vi "ScopeGUI.vi"() -> ()   [LabVIEW 2019]
uses:
  Scope Driver/Typedef/TimeSetting.ctl
  Scope Driver/Typedef/RangeSetting.ctl
  Typedef/Message Format.ctl
  Typedef/Scope Action.ctl
  Typedef/Consumer Loop Data.ctl
  Scope Driver/Typedef/Vertical Settings.ctl
  Scope Driver/Typedef/Channel Selection.ctl
  Scope Driver/Typedef/Coupling.ctl
  Scope Driver/Typedef/TriggerData.ctl
  Scope Driver/Typedef/Edge.ctl
  Scope Driver/Typedef/Horizontal Settings.ctl
  Scope Driver/Typedef/Metadata/[Meta]SetupInfoH.ctl
  Scope Driver/Typedef/Metadata/[Meta]SetupInfoV.ctl
  Scope Driver/Typedef/Metadata/[Meta]SetupInfoTrigger.ctl
  C:/Program Files (x86)/LabNation/SmartScope/DeviceInterface.dll
  Program Files (x86)/LabNation/SmartScope/DeviceInterface.dll
  Scope Driver/LabNation Scope Driver.lvlib
panel:
  in  "Connect":bool
  in  "Tab Control":enum32{"Waveform", "XY"}(tab)
  out "Scope Display":dbl[][](graph)
  in  "Trigger Level":dbl(slide) scale=-4.0..4.0
  in  "Trigger Hold Off":dbl(slide) scale=-2.5e-05..2.5e-05
  out "XY Graph":T1(graph)
  in  "Stop":bool
  in  "ChB Offset":dbl(slide) scale=-4.0..4.0
  in  "ChB V/div":T2=1.0 caption="Knob" scale=0.02..5.0
  in  "ChA Offset":dbl(slide) scale=-4.0..4.0
  in  "ChA V/div":T2=1.0 caption="Knob" scale=0.02..5.0
  out "Connected":bool
  in  "Time/div":T3=0.01 scale=0.0001..1.0 scale format="%#_8g"
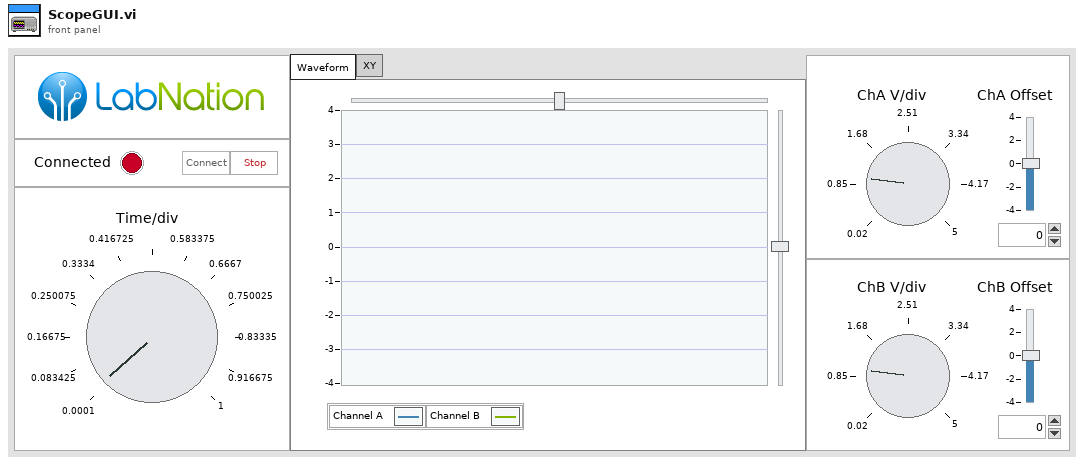
[diagram p1: front panel]
types:
  T1 = cluster{"Waveform Graph":dbl[], "Waveform Graph":dbl[]}
  T2 = typedef "LabNation Scope Driver.lvlib/RangeSetting.ctl" = dbl
  T3 = typedef "LabNation Scope Driver.lvlib/TimeSetting.ctl" = dbl
  T4 = typedef "Message Format.ctl" = cluster{"Action":T5, "Data":variant}
  T5 = typedef "Scope Action.ctl" = enum16{"--- Driver Functions ---", "Init", "SetupV", "SetupTrigger", "SetupH", "AcquireData", "--- UI Setup ---", "UIGraphH", "UIGraphV", "UITrigger", "--- Program Flow ---", "Error Handling", "Stop"}
  T6 = typedef "Consumer Loop Data.ctl" = cluster{"reference":refnum<k24>, "user event out":refnum<user-event>, "Connected?":bool}
  T7 = enum8{"Enabled", "Disabled", "Disabled and Grayed Out"}
  T8 = typedef "LabNation Scope Driver.lvlib/Vertical Settings.ctl" = cluster{"ChannelSelection":T9, "Coupling":T10, "Offset[V]":dbl, "V/div":T2}
  T9 = typedef "LabNation Scope Driver.lvlib/Channel Selection.ctl" = enum16{"chn A", "chn B"}
  T10 = typedef "LabNation Scope Driver.lvlib/Coupling.ctl" = i32
  T11 = typedef "LabNation Scope Driver.lvlib/TriggerData.ctl" = cluster{"Channel":T9, "Edge":T12, "Level[V]":sgl}
  T12 = typedef "LabNation Scope Driver.lvlib/Edge.ctl" = i32
  T13 = typedef "LabNation Scope Driver.lvlib/Horizontal Settings.ctl" = cluster{"Time/div":T3, "Trigger Holdoff":dbl}
  T14 = typedef "LabNation Scope Driver.lvlib/[Meta]SetupInfoH.ctl" = cluster{"xBegin":dbl, "xEnd":dbl}
  T15 = typedef "LabNation Scope Driver.lvlib/[Meta]SetupInfoV.ctl" = cluster{"ChannelSelection":T9, "GraphMin":dbl, "GraphMax":dbl, "OffsetMin":dbl, "OffsetMax":dbl}
  T16 = typedef "LabNation Scope Driver.lvlib/[Meta]SetupInfoTrigger.ctl" = cluster{"Trigger Maximum":dbl, "Trigger Minimum":dbl}
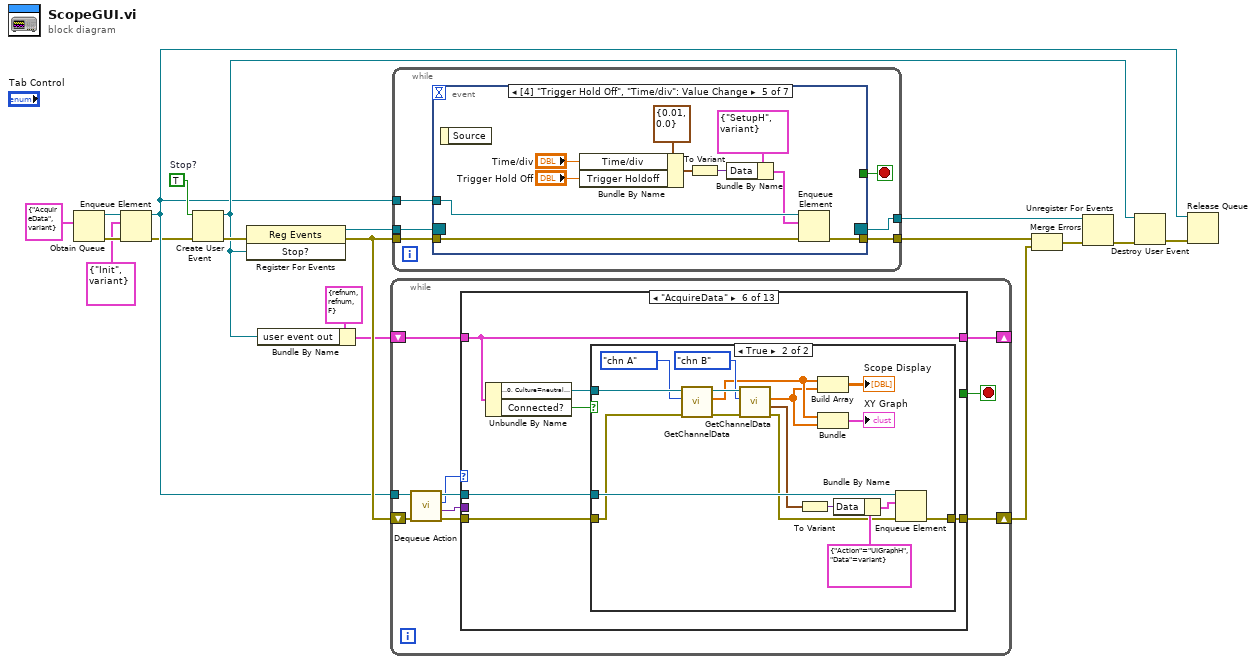
[diagram p0: block diagram]
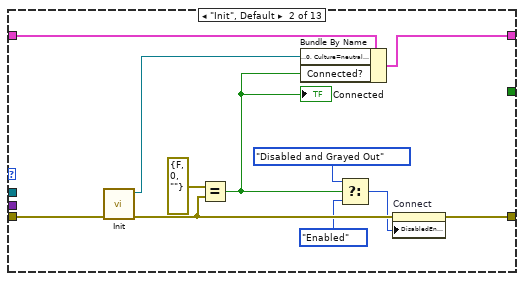
[diagram p3: hidden frame]
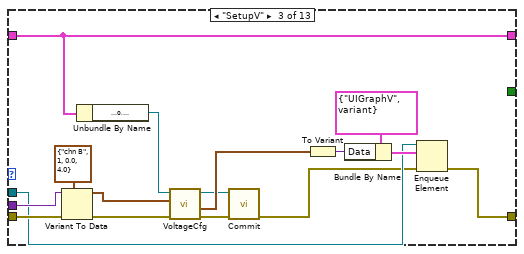
[diagram p4: hidden frame]
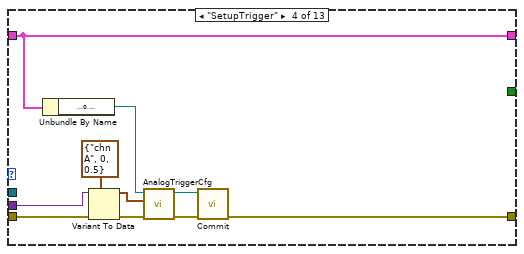
[diagram p5: hidden frame]
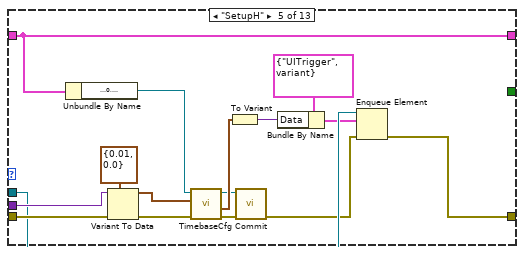
[diagram p6: hidden frame]
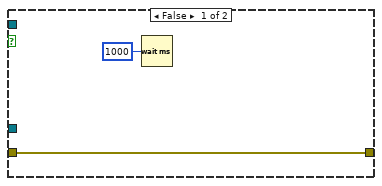
[diagram p7: hidden frame]
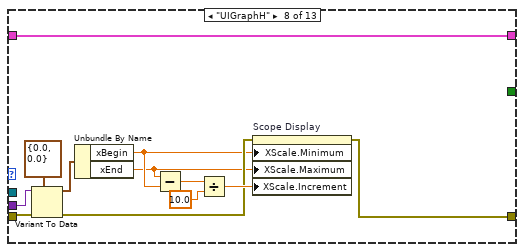
[diagram p9: hidden frame]
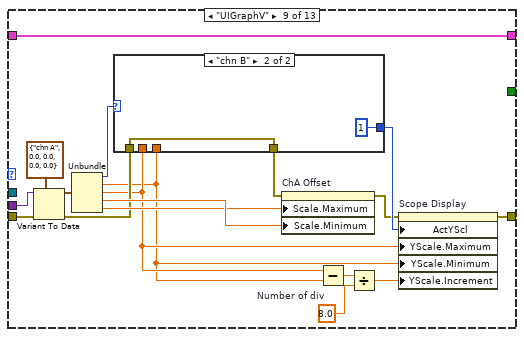
[diagram p10: hidden frame]
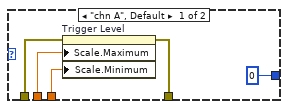
[diagram p11: hidden frame]
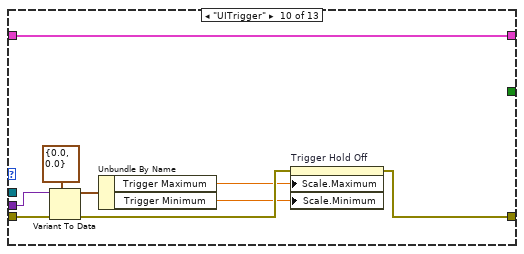
[diagram p12: hidden frame]
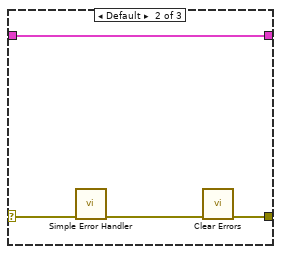
[diagram p15: hidden frame]
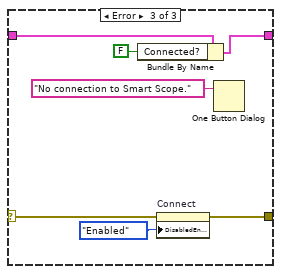
[diagram p16: hidden frame]
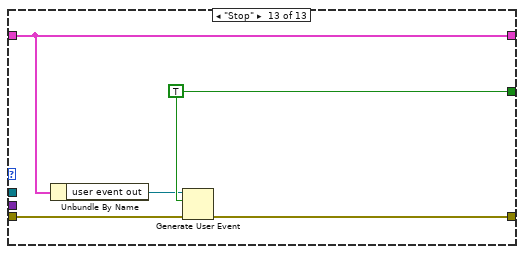
[diagram p17: hidden frame]
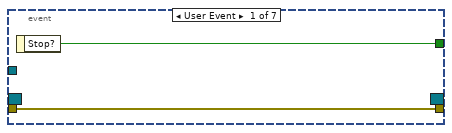
[diagram p18: hidden frame]
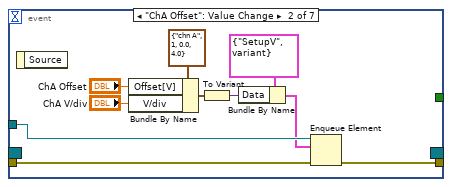
[diagram p19: hidden frame]
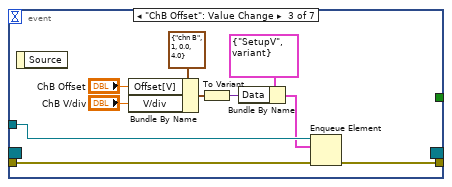
[diagram p20: hidden frame]
diagram:
  w18 = TRUE  # Stop?
  n1 = Obtain Queue(element data type=T4 {"Action"=enum."AcquireData", "Data"=variant}) -> (queue out=w5:refnum<queue>, error out=w2:errorcluster)  [unwired: 4 in, 1 out]
  n2 = Enqueue Element(queue=w5, element=T4 {"Action"=enum."Init", "Data"=variant}, error in (no error)=w2) -> (queue out=w4:refnum<queue>, error out=w3:errorcluster)  [unwired: 1 in, 1 out]
  n3 = Create User Event(user event datatype=w18, error in=w3) -> (user event=w7:refnum<user-event>, error out=w17:errorcluster)
  n4 = register-events(error in=w17, w7) -> (reference out=w19:refnum<event-registration>, error out=w10:errorcluster)  [unwired: 1 in]
  n5 = Bundle By Name(cluster=T6 {"reference"=refnum, "user event out"=refnum, "Connected?"=FALSE}, "user event out"=w7) -> (w6:T6)
  n6 = while {
    tunnel: w4 -> [w28]
    shift-right: [w24] -> w9
    shift-left: w10 -> [w29]
    shift-right: [w21] -> _
    shift-left: w6 -> [w22]
    stop <- w23 stop-if-true
    n7 = call "Dequeue Action.vi"("error in (no error)"=w29, "Queue in"=w28) -> ("error out"=w25:errorcluster, "Data"=w20:variant, "Action"=w26:T5, "Queue out"=w27:refnum<queue>)  [unwired: 6 in]
    n8 = case shown="\"AcquireData\"" w26 {
      tunnel: w27 -> [_ _ w45 _ w75 w86 _ _ _ _ _ _ _]
      tunnel: w20 -> [_ _ w53 w63 w80 _ _ w119 w139 w154 _ _ _]
      tunnel: w25 -> [w30 w42 w58 w68 w81 w90 w110 w121 w140 w157 w158 w162 w181]
      tunnel: w22 -> [w31 w41 w56 w65 w84 w88 w111 w112 w141 w149 w159 w160 w177]
      tunnel: [w30 w36 w46 w60 w74 w87 w110 w116 w132 w155 w158 w163 w180] -> w24
      tunnel: [_ _ _ _ _ _ _ _ _ _ _ _ w179] -> w23
      tunnel: [w31 w40 w56 w65 w84 w88 w111 w112 w141 w149 w159 w161 w177] -> w21
      frame "--- Driver Functions ---" {
      }
      frame "Init", Default {
        n9 = call "Init.vi"("error in (no error)"=w42) -> ("error out"=w37:errorcluster, "reference out"=w39:refnum<k24>)  [unwired: 9 in]
        n10 = Equal?(x=errorcluster {"status"=FALSE, "code"=0, "source"=""}, y=w37) -> (x = y?=w35:bool)
        "Connected" <- w35
        n11 = Bundle By Name(cluster=w41, "reference"=w39, "Connected?"=w35) -> (w40:T6)
        n12 = Select(t=T7."Disabled and Grayed Out" ("Disabled"), s=w35, f=T7."Enabled" ("Disabled")) -> (s? t:f=w32:T7)
        n13 = property on="Connect" class="Bool"(error in=w37, "DisabledEnum"=w32) -> (error out=w36:errorcluster)  [unwired: 1 in, 1 out]
      }
      frame "SetupV" {
        n14 = Variant To Data(error in=w58, type=T8 {"ChannelSelection"=enum."chn B", "Coupling"=1, "Offset[V]"=0.0, "V/div"=4.0} ("Vertical Settings"), Variant=w53) -> (data=w52:T8, error out=w55:errorcluster)
        n15 = Unbundle By Name(w56) -> ("reference"=w57:refnum<k24>)
        n16 = call "VoltageCfg.vi"("error in (no error)"=w55, "Vertical Settings"=w52, "reference in"=w57) -> ("error out"=w47:errorcluster, "Setup Info Vertical"=w48:T15, "reference out"=w43:refnum<k24>)  [unwired: 6 in]
        n17 = call "Commit.vi"("error in (no error)"=w47, "reference in"=w43) -> ("error out"=w44:errorcluster)  [unwired: 8 in, 1 out]
        n18 = To Variant(anything=w48) -> (Variant=w51:variant)
        n19 = Bundle By Name(cluster=T4 {"Action"=enum."UIGraphV", "Data"=variant} ("element"), "Data"=w51) -> (w50:T4)
        n20 = Enqueue Element(queue=w45, element=w50, error in (no error)=w44) -> (error out=w46:errorcluster)  [unwired: 1 in, 2 out]
      }
      frame "SetupTrigger" {
        n21 = Unbundle By Name(w65) -> ("reference"=w66:refnum<k24>)
        n22 = Variant To Data(error in=w68, type=T11 {"Channel"=enum."chn A", "Edge"=0, "Level[V]"=0.5} ("Trigger Config"), Variant=w63) -> (data=w61:T11, error out=w64:errorcluster)
        n23 = call "AnalogTriggerCfg.vi"("error in (no error)"=w64, "Trigger Config"=w61, "reference in"=w66) -> ("error out"=w67:errorcluster, "reference out"=w59:refnum<k24>)  [unwired: 7 in]
        n24 = call "Commit.vi"("error in (no error)"=w67, "reference in"=w59) -> ("error out"=w60:errorcluster)  [unwired: 8 in, 1 out]
      }
      frame "SetupH" {
        n25 = Unbundle By Name(w84) -> ("reference"=w83:refnum<k24>)
        n26 = Variant To Data(error in=w81, type=T13 {"Time/div"=0.01, "Trigger Holdoff"=0.0} ("Horizontal Settings"), Variant=w80) -> (data=w78:T13, error out=w82:errorcluster)
        n27 = call "TimebaseCfg.vi"("error in (no error)"=w82, "Horizontal Settings"=w78, "reference in"=w83) -> ("error out"=w76:errorcluster, "Setup Info Horizontal"=w77:T16, "reference out"=w69:refnum<k24>)  [unwired: 6 in]
        n28 = To Variant(anything=w77) -> (Variant=w71:variant)
        n29 = call "Commit.vi"("error in (no error)"=w76, "reference in"=w69) -> ("error out"=w70:errorcluster)  [unwired: 8 in, 1 out]
        n30 = Bundle By Name(cluster=T4 {"Action"=enum."UITrigger", "Data"=variant} ("element"), "Data"=w71) -> (w72:T4)
        n31 = Enqueue Element(queue=w75, element=w72, error in (no error)=w70) -> (error out=w74:errorcluster)  [unwired: 1 in, 2 out]
      }
      frame "AcquireData" {
        n32 = Unbundle By Name(w88) -> ("reference"=w89:refnum<k24>, "Connected?"=w85:bool)
        n33 = case shown="True" w85 {
          tunnel: w90 -> [w91 w97]
          tunnel: w89 -> [_ w109]
          tunnel: [w91 w102] -> w87
          tunnel: w86 -> [_ w101]
          frame False {
            n34 = Wait (ms)(milliseconds to wait=u32 1000) -> ()  [unwired: 1 out]
          }
          frame True {
            n35 = call "GetChannelData.vi"("error in (no error)"=w97, "ChannelSelection"=Channel_Selection."chn A", "reference in"=w109) -> ("error out"=w108:errorcluster, "Waveform Graph"=w95:dbl[], "reference out"=w107:refnum<k24>)  [unwired: 5 in, 1 out]
            n36 = call "GetChannelData.vi"("error in (no error)"=w108, "ChannelSelection"=Channel_Selection."chn B", "reference in"=w107) -> ("error out"=w96:errorcluster, "[Meta]Setup Info H"=w99:T14, "Waveform Graph"=w94:dbl[])  [unwired: 5 in, 1 out]
            n37 = To Variant(anything=w99) -> (Variant=w98:variant)
            n38 = Build Array(w95, w94) -> (→"Scope Display":dbl[][])
            n39 = Bundle("Waveform Graph"=w95, "Waveform Graph"=w94) -> (→"XY Graph":T1)  [unwired: 1 in]
            n40 = Bundle By Name(cluster=T4 {"Action"=enum."UIGraphH", "Data"=variant} ("element"), "Data"=w98) -> (w103:T4)
            n41 = Enqueue Element(queue=w101, element=w103, error in (no error)=w96) -> (error out=w102:errorcluster)  [unwired: 1 in, 2 out]
          }
        }
      }
      frame "--- UI Setup ---" {
      }
      frame "UIGraphH" {
        n42 = Variant To Data(error in=w121, type=T14 {"xBegin"=0.0, "xEnd"=0.0} ("[Meta]Setup Info H"), Variant=w119) -> (data=w115:T14, error out=w117:errorcluster)
        n43 = Unbundle By Name(w115) -> ("xBegin"=w114:dbl, "xEnd"=w113:dbl)
        n44 = Subtract(x=w113, y=w114) -> (x-y=w122:dbl)
        n45 = Divide(x=w122, y=10.0) -> (x/y=w123:dbl)
        n46 = property on="Scope Display" class="WFGraph (strict)"(error in=w117, "XScale.Minimum"=w114, "XScale.Maximum"=w113, "XScale.Increment"=w123) -> (error out=w116:errorcluster)  [unwired: 1 in, 1 out]
      }
      frame "UIGraphV" {
        w131 = 8.0  # Number of div
        n47 = Variant To Data(error in=w140, type=T15 {"ChannelSelection"=enum."chn A", "GraphMin"=0.0, "GraphMax"=0.0, "OffsetMin"=0.0, "OffsetMax"=0.0} ("Setup Info Vertical"), Variant=w139) -> (data=w137:T15, error out=w128:errorcluster)
        n48 = Unbundle(w137) -> ("ChannelSelection"=w136:T9, "GraphMin"=w124:dbl, "GraphMax"=w125:dbl, "OffsetMin"=w130:dbl, "OffsetMax"=w129:dbl)
        n49 = case shown="\"chn B\"" w136 {
          tunnel: [0 ("Active Y Scale") 1 ("Active Y Scale")] -> w133
          tunnel: w128 -> [w145 w148]
          tunnel: w125 -> [w144 _]
          tunnel: w124 -> [w143 _]
          tunnel: [w142 w148] -> w127
          frame "chn A", Default {
            n50 = property on="Trigger Level" class="Slide (strict)"(error in=w145, "Scale.Maximum"=w144, "Scale.Minimum"=w143) -> (error out=w142:errorcluster)  [unwired: 1 in, 1 out]
          }
          frame "chn B" {
          }
        }
        n51 = property on="ChA Offset" class="Slide (strict)"(error in=w127, "Scale.Maximum"=w129, "Scale.Minimum"=w130) -> (error out=w126:errorcluster)  [unwired: 1 in, 1 out]
        n52 = Subtract(x=w125, y=w124) -> (x-y=w134:dbl)
        n53 = Divide(x=w134, y=w131) -> (x/y=w135:dbl)
        n54 = property on="Scope Display" class="WFGraph (strict)"(error in=w126, "ActYScl"=w133, "YScale.Maximum"=w125, "YScale.Minimum"=w124, "YScale.Increment"=w135) -> (error out=w132:errorcluster)  [unwired: 1 in, 1 out]
      }
      frame "UITrigger" {
        n55 = Variant To Data(error in=w157, type=T16 {"Trigger Maximum"=0.0, "Trigger Minimum"=0.0} ("Setup Info Horizontal"), Variant=w154) -> (data=w152:T16, error out=w156:errorcluster)
        n56 = Unbundle By Name(w152) -> ("Trigger Maximum"=w151:dbl, "Trigger Minimum"=w150:dbl)
        n57 = property on="Trigger Hold Off" class="Slide (strict)"(error in=w156, "Scale.Maximum"=w151, "Scale.Minimum"=w150) -> (error out=w155:errorcluster)  [unwired: 1 in, 1 out]
      }
      frame "--- Program Flow ---" {
      }
      frame "Error Handling" {
        n58 = case shown="No Error" w162 {
          selector: w162 -> [w165 w167 w170]
          tunnel: [w165 w169 w171] -> w163
          tunnel: [w164 w166 w174] -> w161
          tunnel: w160 -> [w164 w166 w175]
          frame No Error {
          }
          frame Default {
            n59 = call <vilib>:"Simple Error Handler.vi"("error in (no error)"=w167) -> ("error out"=w168:errorcluster)  [unwired: 4 in, 4 out]
            n60 = call <vilib>:"Clear Errors.vi"("error in (no error)"=w168) -> ("error out"=w169:errorcluster)  [unwired: 5 in, 1 out]
          }
          frame Error {
            n61 = Bundle By Name(cluster=w175, "Connected?"=FALSE) -> (w174:T6)
            n62 = property on="Connect" class="Bool"(error in=w170, "DisabledEnum"=T7."Enabled" ("Disabled")) -> (error out=w171:errorcluster)  [unwired: 1 in, 1 out]
            n63 = One Button Dialog(message="No connection to Smart Scope.") -> ()  [unwired: 1 in, 1 out]
          }
        }
      }
      frame "Stop" {
        w179 = TRUE ("event data")
        n64 = Unbundle By Name(w177) -> ("user event out"=w178:refnum<user-event>)
        n65 = Generate User Event(user event=w178, event data cluster=w179, error in=w181) -> (error out=w180:errorcluster)  [unwired: 1 in, 1 out]
      }
    }
  }
  n66 = while {
    tunnel: w19 -> [w187]
    tunnel: [w186] -> w16
    tunnel: w10 -> [w185]
    tunnel: [w183] -> w14
    tunnel: w4 -> [w182]
    stop <- w184 stop-if-true
    n67 = event shown="[4] \"Trigger Hold Off\", \"Time/div\": Value Change" {
      selector: w187 -> [_ _ _ _ _ _ _]
      dyn-events: [_ _ _ _ _ _ _] -> w183
      timeout: _ -> [_ _ _ _ _ _ _]
      tunnel: [w189 w197 w207 w216 w226 w230 w235] -> w186
      tunnel: w185 -> [w189 w198 w208 w217 w227 w232 w234]
      tunnel: [w188 _ _ _ _ _ _] -> w184
      tunnel: w182 -> [_ w199 w209 w218 w228 w231 w233]
      event User Event {
        n68 = event-data() -> ("Stop?"=w188:bool)  [unwired: 1 in]
      }
      event "ChA Offset": Value Change {
        n69 = event-data() -> ()  [unwired: 1 in, 1 out]
        n70 = Bundle By Name(cluster=T8 {"ChannelSelection"=enum."chn A", "Coupling"=1, "Offset[V]"=0.0, "V/div"=4.0} ("Vertical Settings"), "Offset[V]"="ChA Offset", "V/div"="ChA V/div") -> (w194:T8)
        n71 = To Variant(anything=w194) -> (Variant=w190:variant)
        n72 = Bundle By Name(cluster=T4 {"Action"=enum."SetupV", "Data"=variant} ("element"), "Data"=w190) -> (w191:T4)
        n73 = Enqueue Element(queue=w199, element=w191, error in (no error)=w198) -> (error out=w197:errorcluster)  [unwired: 1 in, 2 out]
      }
      event "ChB Offset": Value Change {
        n74 = event-data() -> ()  [unwired: 1 in, 1 out]
        n75 = Bundle By Name(cluster=T8 {"ChannelSelection"=enum."chn B", "Coupling"=1, "Offset[V]"=0.0, "V/div"=4.0} ("Vertical Settings"), "Offset[V]"="ChB Offset", "V/div"="ChB V/div") -> (w206:T8)
        n76 = To Variant(anything=w206) -> (Variant=w203:variant)
        n77 = Bundle By Name(cluster=T4 {"Action"=enum."SetupV", "Data"=variant} ("element"), "Data"=w203) -> (w204:T4)
        n78 = Enqueue Element(queue=w209, element=w204, error in (no error)=w208) -> (error out=w207:errorcluster)  [unwired: 1 in, 2 out]
      }
      event "Trigger Level": Value Change {
        n79 = event-data() -> ()  [unwired: 1 in, 1 out]
        n80 = Bundle By Name(cluster=T11 {"Channel"=enum."chn A", "Edge"=0, "Level[V]"=0.5} ("Trigger Config"), "Level[V]"="Trigger Level") -> (w215:T11)
        n81 = To Variant(anything=w215) -> (Variant=w212:variant)
        n82 = Bundle By Name(cluster=T4 {"Action"=enum."SetupTrigger", "Data"=variant} ("element"), "Data"=w212) -> (w213:T4)
        n83 = Enqueue Element(queue=w218, element=w213, error in (no error)=w217) -> (error out=w216:errorcluster)  [unwired: 1 in, 2 out]
      }
      event "Trigger Hold Off": Value Change {
        n84 = event-data() -> ()  [unwired: 1 in, 1 out]
        n85 = Bundle By Name(cluster=T13 {"Time/div"=0.01, "Trigger Holdoff"=0.0} ("Horizontal Settings"), "Time/div"="Time/div", "Trigger Holdoff"="Trigger Hold Off") -> (w225:T13)
        n86 = To Variant(anything=w225) -> (Variant=w222:variant)
        n87 = Bundle By Name(cluster=T4 {"Action"=enum."SetupH", "Data"=variant} ("element"), "Data"=w222) -> (w223:T4)
        n88 = Enqueue Element(queue=w228, element=w223, error in (no error)=w227) -> (error out=w226:errorcluster)  [unwired: 1 in, 2 out]
      }
      event "Stop": Value Change {
        n89 = event-data() -> ()  [unwired: 1 in, 1 out]
        n90 = Enqueue Element(queue=w231, element=T4 {"Action"=enum."Stop", "Data"=variant}, error in (no error)=w232) -> (error out=w230:errorcluster)  [unwired: 1 in, 2 out]
      }
      event "Connect": Value Change {
        n91 = event-data() -> ()  [unwired: 1 in, 1 out]
        n92 = Enqueue Element(queue=w233, element=T4 {"Action"=enum."Init", "Data"=variant}, error in (no error)=w234) -> (error out=w235:errorcluster)  [unwired: 1 in, 2 out]
      }
    }
  }
  n93 = Merge Errors(w16, w9) -> (w15:errorcluster)
  n94 = Unregister For Events(event registration refnum=w14, error in=w15) -> (error out=w13:errorcluster)
  n95 = Destroy User Event(user event=w7, error in=w13) -> (error out=w12:errorcluster)
  n96 = Release Queue(queue=w4, error in (no error)=w12) -> ()  [unwired: 1 in, 3 out]
